vi "vücut kitle indeksi hesaplama.vi"() -> ()   [LabVIEW 2017]
uses:
  <vilib>/LabVIEW Interface for Arduino/Type Defs/LCD Pin Config 4 bit.ctl
  <vilib>/LabVIEW Interface for Arduino/LabVIEW Interface for Arduino.lvlib
panel:
  in  "stop":bool
  in  "Row":u8
  in  "Column":u8
  in  "LCD Pin Config 4 Bit":T1={"RS"=12, "RW"=255, "Enable"=11, "D4"=5, "D5"=4, "D6"=3, "D7"=2, "LCD"=7}
  in  "VISA resource":refnum<visa-resource-name>
  in  "OK Button":bool
  out "vücut kitle indeksi durumunuz":string
  out "vücut kitle indeksiniz":dbl
  in  "boyunuz metre cinsinden giriniz":dbl
  in  "kilonuzu kg cinsinden giriniz":dbl
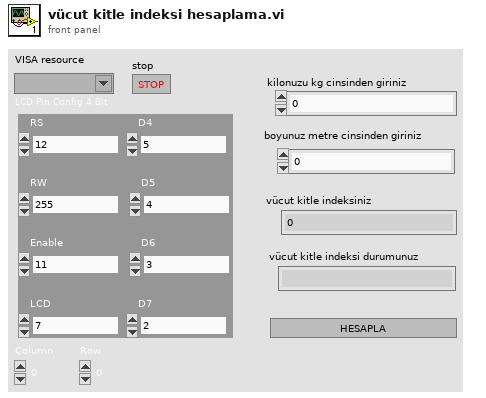
[diagram p1: front panel]
types:
  T1 = typedef "LabVIEW Interface for Arduino.lvlib/LCD Pin Config 4 bit.ctl" = cluster{"RS":u8, "RW":u8, "Enable":u8, "D4":u8, "D5":u8, "D6":u8, "D7":u8, "LCD":u8}
  T2 = typedef "LabVIEW Interface for Arduino.lvlib/Arduino Resource.ctl" = cluster{"VISA resource":refnum<visa-resource-name>, "Board Type":T3, "Connection Type":enum8{"USB / Serial"}, "Bytes Per Packet (15)":u8}
  T3 = typedef "LabVIEW Interface for Arduino.lvlib/Board Type.ctl" = enum16{"Uno", "Dimuelanove w/Atmega 328", "Mega 2560"}
  T4 = enum8{"String", "Binary", "Decimal", "Octal", "Hexadecimal"}
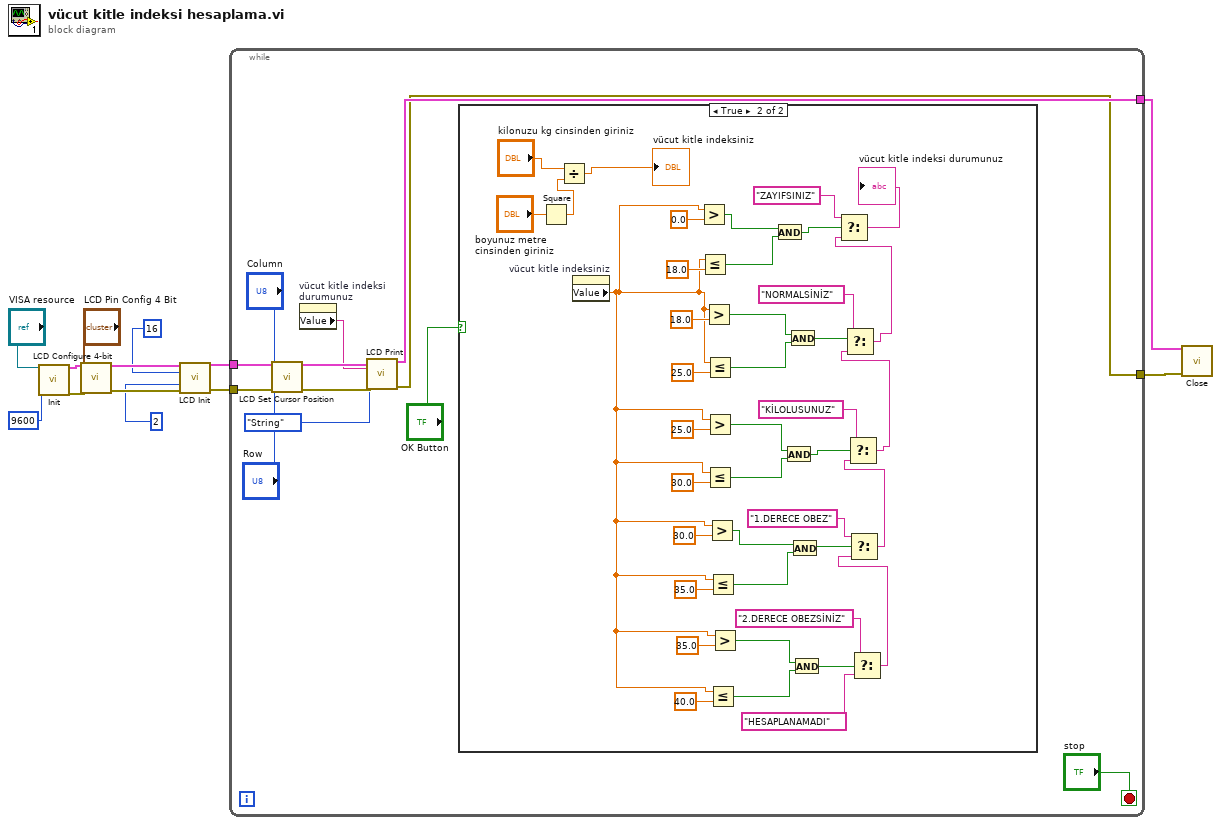
[diagram p0: block diagram]
diagram:
  n1 = call <vilib>:"Init.vi"("VISA resource"="VISA resource", "Baud Rate (115200)"=u32 9600) -> ("Arduino Resource"=w13:T2, "error out"=w12:errorcluster)  [unwired: 16 in]
  n2 = call <vilib>:"LCD Configure 4-bit.vi"("Arduino Resource"=w13, "LCD Pin Config 4 Bit"="LCD Pin Config 4 Bit", "error in"=w12) -> ("Arduino Resource"=w11:T2, "error out"=w10:errorcluster)  [unwired: 11 in]
  n3 = call <vilib>:"LCD Init.vi"("Arduino Resource"=w11, "Columns"=u8 16, "Rows"=u8 2, "error in"=w10) -> ("Arduino Resource"=w5:T2, "error out"=w4:errorcluster)  [unwired: 10 in]
  n4 = while {
    tunnel: w5 -> [w22]
    tunnel: w4 -> [w21]
    tunnel: [w15] -> w1
    tunnel: [w14] -> w2
    stop <- "stop" stop-if-true
    n5 = call <vilib>:"LCD Set Cursor Position.vi"("Arduino Resource"=w22, "Column"="Column", "Row"="Row", "error out"=w21) -> ("Arduino Resource"=w24:T2, "error out"=w23:errorcluster)  [unwired: 10 in]
    n6 = property on="vücut kitle indeksi durumunuz" class="Str"() -> ("Value"=w17:string)  [unwired: 2 in, 2 out]
    n7 = call <vilib>:"LCD Print.vi"("Arduino Resource"=w24, "Data"=w17, "Base (String)"=T4."String", "error out"=w23) -> ("Arduino Resource"=w15:T2, "error out"=w14:errorcluster)  [unwired: 10 in]
    n8 = case shown="True" "OK Button" {
      frame False {
      }
      frame True {
        n9 = Square(x="boyunuz metre cinsinden giriniz") -> (x^2=w65:dbl)
        n10 = Divide(x="kilonuzu kg cinsinden giriniz", y=w65) -> (x/y=→"vücut kitle indeksiniz":dbl)
        n11 = property on="vücut kitle indeksiniz" class="DigNum (strict)"() -> ("Value"=w38:dbl)  [unwired: 2 in, 2 out]
        n12 = Greater?(x=w38, y=0.0) -> (0:w52:bool)
        n13 = Less Or Equal?(x=w38, y=18.0) -> (x <= y?=w53:bool)
        n14 = Greater?(x=w38, y=18.0) -> (0:w54:bool)
        n15 = Less Or Equal?(x=w38, y=25.0) -> (x <= y?=w55:bool)
        n16 = Greater?(x=w38, y=25.0) -> (0:w57:bool)
        n17 = Less Or Equal?(x=w38, y=30.0) -> (x <= y?=w56:bool)
        n18 = Greater?(x=w38, y=30.0) -> (0:w37:bool)
        n19 = Less Or Equal?(x=w38, y=35.0) -> (x <= y?=w36:bool)
        n20 = Less Or Equal?(x=w38, y=40.0) -> (x <= y?=w34:bool)
        n21 = Greater?(x=w38, y=35.0) -> (0:w35:bool)
        n22 = And(x=w52, y=w53) -> (x .and. y?=w49:bool)
        n23 = And(x=w57, y=w56) -> (x .and. y?=w51:bool)
        n24 = And(x=w54, y=w55) -> (x .and. y?=w50:bool)
        n25 = And(x=w37, y=w36) -> (x .and. y?=w32:bool)
        n26 = And(x=w35, y=w34) -> (x .and. y?=w30:bool)
        n27 = Select(t="2.DERECE OBEZSİNİZ" ("String"), s=w30, f="HESAPLANAMADI") -> (s? t:f=w28:string)
        n28 = Select(t="1.DERECE OBEZ" ("String"), s=w32, f=w28) -> (s? t:f=w31:string)
        n29 = Select(t="KİLOLUSUNUZ" ("String"), s=w51, f=w31) -> (s? t:f=w44:string)
        n30 = Select(t="NORMALSİNİZ" ("String"), s=w50, f=w44) -> (s? t:f=w45:string)
        n31 = Select(t="ZAYIFSINIZ" ("String"), s=w49, f=w45) -> (s? t:f=→"vücut kitle indeksi durumunuz":string)
      }
    }
  }
  n32 = call <vilib>:"Close.vi"("Arduino Resource"=w1, "error in"=w2) -> ()  [unwired: 13 in, 1 out]
